vi "create folder with deletion.vi"(8 "error in (no error)":errorcluster, 10 "Folder Name":string, 11 "Root path":path) -> (0 "error out":errorcluster, 3 "created path":path)   [LabVIEW 2022 SP3]
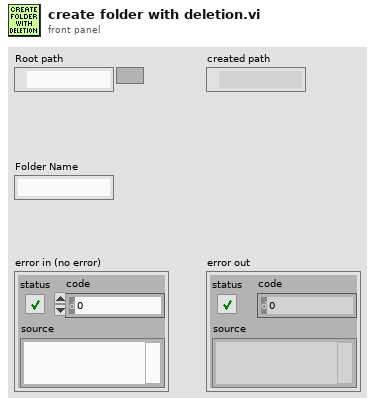
[diagram p1: front panel]
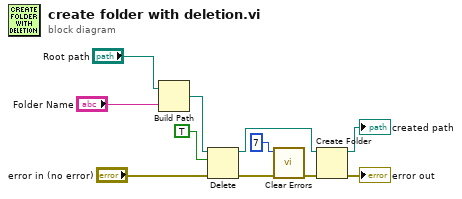
[diagram p0: block diagram]
diagram:
  n1 = Build Path(base path="Root path", name or relative path="Folder Name") -> (appended path=w5:path)
  n2 = Delete(path (use dialog)=w5, entire hierarchy (F)=TRUE, error in="error in (no error)") -> (deleted path=w8:path, error out=w10:errorcluster)  [unwired: 2 in, 1 out]
  n3 = call <vilib>:"Clear Errors.vi"("error in (no error)"=w10, "specific error code to clear (0: all)"=7) -> ("error out"=w11:errorcluster)  [unwired: 4 in, 1 out]
  n4 = Create Folder(path (use dialog)=w8, error in=w11) -> (created path=→"created path":path, error out=→"error out":errorcluster)  [unwired: 1 in, 1 out]
